vi "Read configuration.vi"(8 "error in (no error)":errorcluster, 11 "Device Channel in":refnum<class "FPGA Channel.lvclass">) -> (0 "error out":errorcluster, 2 "configuration":refnum<class "CEF_serializable configuration.lvclass">, 3 "Device Channel out":refnum<class "FPGA Channel.lvclass">)   [LabVIEW 2025, in "FPGA.lvlib" / "FPGA Channel.lvclass"]
uses:
  FPGA Channel.lvclass
  Users/Public/Documents/Sandia National Labs/TSS Plugin/CEF.lvlibp/serializable configuration/CEF_serializable configuration.lvclass
  FPGA Channel.lvclass/FPGA Channel.ctl
  FPGA Channel configuration/FPGA Channel configuration.lvclass
  C:/Users/Public/Documents/Sandia National Labs/TSS Plugin/CEF.lvlibp/serializable configuration/CEF_serializable configuration.lvclass
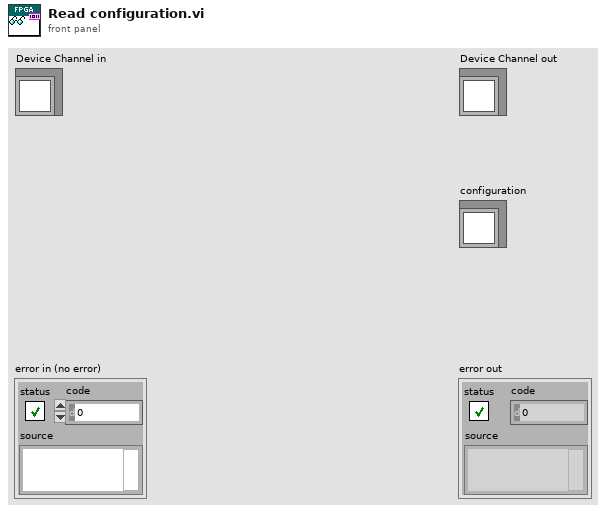
[diagram p1: front panel]
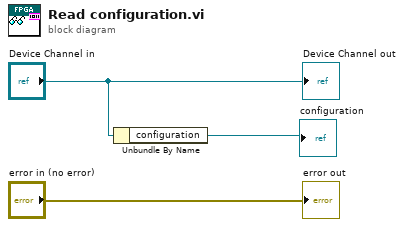
[diagram p0: block diagram]
diagram:
  n1 = Unbundle By Name("Device Channel in") -> ("configuration"=→"configuration":refnum<class "FPGA Channel configuration.lvclass">)
  "error out" <- "error in (no error)"
  "Device Channel out" <- "Device Channel in"
